vi "Read-n-Update INI File.vi"(8 "error in (no error)":errorcluster) -> (0 "error out":errorcluster, 3 "Config Data Out":cluster{"Company":string, "Author":string})   [LabVIEW 2014]
uses:
  <vilib>/Utility/config.llb/Read Key (String).vi
  <vilib>/Utility/config.llb/NI_LVConfig.lvlib
panel:
  out "appended path":path
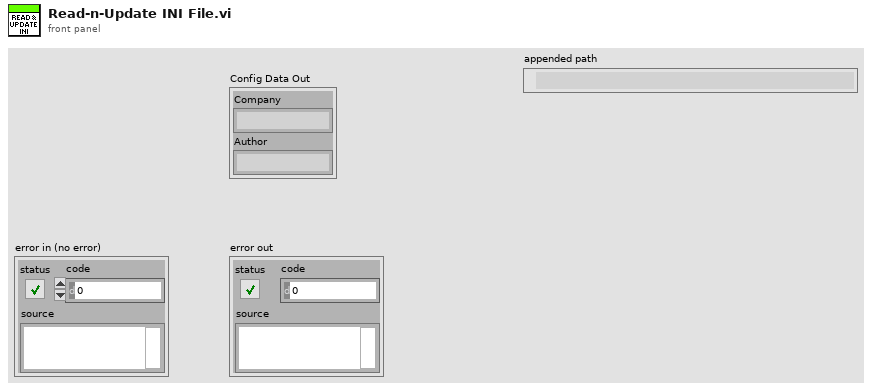
[diagram p1: front panel]
types:
  T1 = typedef "NI_LVConfig.lvlib/Config Data RefNum.ctl" = refnum<k1>
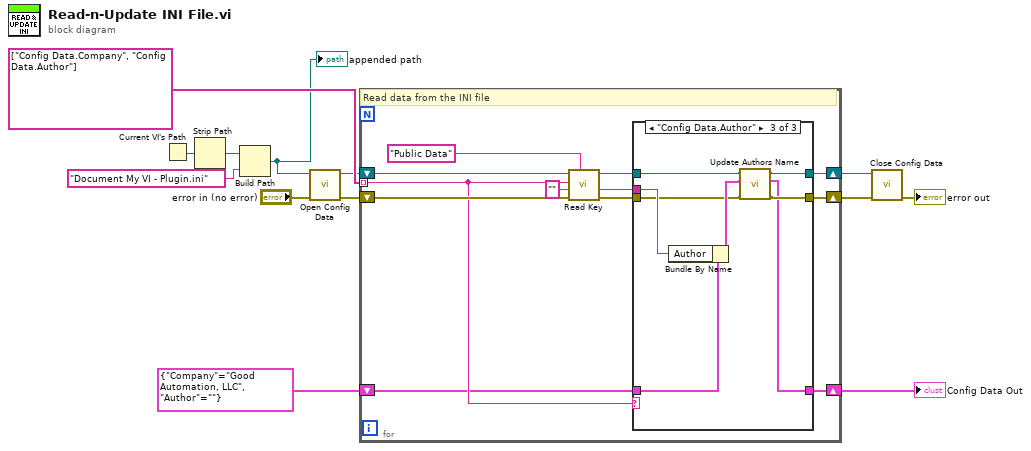
[diagram p0: block diagram]
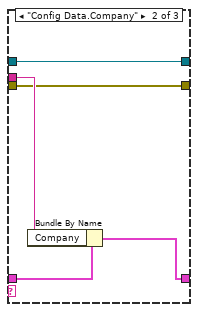
[diagram p3: hidden frame]
diagram:
  n1 = Current VI's Path() -> (path=w12:path)
  n2 = Strip Path(path=w12) -> (stripped path=w2:path)  [unwired: 1 out]
  n3 = Build Path(base path=w2, name or relative path="Document My VI - Plugin.ini") -> (appended path=w5:path)
  "appended path" <- w5
  n4 = call <vilib>:"Open Config Data.vi"("error in (no error)"="error in (no error)", "configuration file path"=w5) -> ("error out"=w6:errorcluster, "refnum"=w8:T1)  [unwired: 7 in, 1 out]
  n5 = for {
    shift-right: [w17] -> w9
    shift-left: w8 -> [w23]
    shift-right: [w19] -> w7
    shift-left: w6 -> [w25]
    tunnel: string[] ["Config Data.Company", "Config Data.Author"] -> [w22] mode=indexing
    shift-right: [w15] -> w3
    shift-left: cluster{"Company":string, "Author":string} {"Company"="Good Automation, LLC", "Author"=""} ("Config Data In") -> [w16]
    # "Read data from the INI file"
    n6 = call-poly <vilib>:"Read Key.vi"("section"="Public Data", "error in (no error)"=w25, "default value"="", "key"=w22, "refnum"=w23) -> ("error out"=w20:errorcluster, "value"=w21:string, "refnum out"=w18:T1)  [unwired: 3 in, 1 out]
    n7 = case shown="\"Config Data.Author\"" w22 {
      tunnel: w16 -> [w26 w33 w41]
      tunnel: [w26 w29 w34] -> w15
      tunnel: w21 -> [_ w32 w40]
      tunnel: w20 -> [w27 w31 w38]
      tunnel: w18 -> [w28 w30 w35]
      tunnel: [w27 w31 w37] -> w19
      tunnel: [w28 w30 w36] -> w17
      frame "False", Default {
      }
      frame "Config Data.Company" {
        n8 = Bundle By Name(cluster=w33, "Company"=w32) -> (w29:cluster{"Company":string, "Author":string})
      }
      frame "Config Data.Author" {
        n9 = Bundle By Name(cluster=w41, "Author"=w40) -> (w39:cluster{"Company":string, "Author":string})
        n10 = call "Update Authors Name.vi"("INI File Ref In"=w35, "Config Data In"=w39, "error in"=w38) -> ("INI File Ref Out"=w36:T1, "Config Data Out"=w34:cluster{"Company":string, "Author":string}, "error out"=w37:errorcluster)  [unwired: 5 in]
      }
    }
  }
  "Config Data Out" <- w3
  n11 = call <vilib>:"Close Config Data.vi"("error in (no error)"=w7, "refnum"=w9) -> ("error out"=→"error out":errorcluster)  [unwired: 8 in, 1 out]
